vi "HIOKI PW3390 Acquisition Software Trigger.vi"() -> ()   [LabVIEW 2009]
doc: "When each time pushing the trigger button, outputs the specified measurement data."
uses:
  <instrlib>/PW3390/Common/_Initialize/HIOKI PW3390 Initialize LAN.vi
  <instrlib>/PW3390/Common/_Initialize/HIOKI PW3390 Initialize RS-232C.vi
panel:
  out "Selected Item out":string[](array[string])
  in  "Item":T1(array[cluster])=[{"Item"=enum."Urms", "Ch(0:Ch1)"=enum."1"}, {"Item"=enum."Urms", "Ch(0:Ch1)"=enum."2"}, {"Item"=enum."Urms", "Ch(0:Ch1)"=enum."3"}, {"Item"=enum."Urms", "Ch(0:Ch1)"=enum."4"}]
  out "Data out":dbl[](array[numeric])
  out "error out":errorcluster
  in  "Communication Interface":enum16{"LAN", "RS-232C"}(ring)
  in  "COM Port":refnum<visa-resource-name>="COM1"
  in  "baud rate (38400bps)":u32=38400
  in  "IP Address":string="192.168.1.1"
  in  "Trigger":bool
  in  "Stop":bool
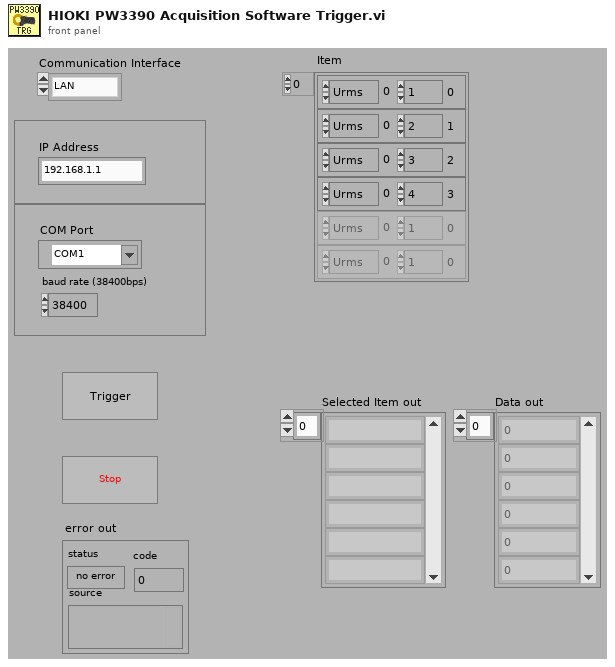
[diagram p1: front panel]
types:
  T1 = cluster{"Item":enum16{"Urms", "Umn", "Uac", "Udc", "Ufnd", "Upk+", "Upk-", "Uthd", "Urf", "Uunb", "Irms", "Imn", "Iac", "Idc", "Ifnd", "Ipk+", "Ipk-", "Ithd", "Irf", "Iunb", "P", "S", "Q", "PF", "DEG U", "DEG I", "DEG P", "f", "EFFI", "LOSS", "IH+", "IH-", "IH", "WP+", "WP-", "WP", "CH A", "CH B", "Pm", "Slip", "Laptime", "Laptime(ms)"}, "Ch(0:Ch1)":enum16{"1", "2", "3", "4", "12", "34", "123"}}[]
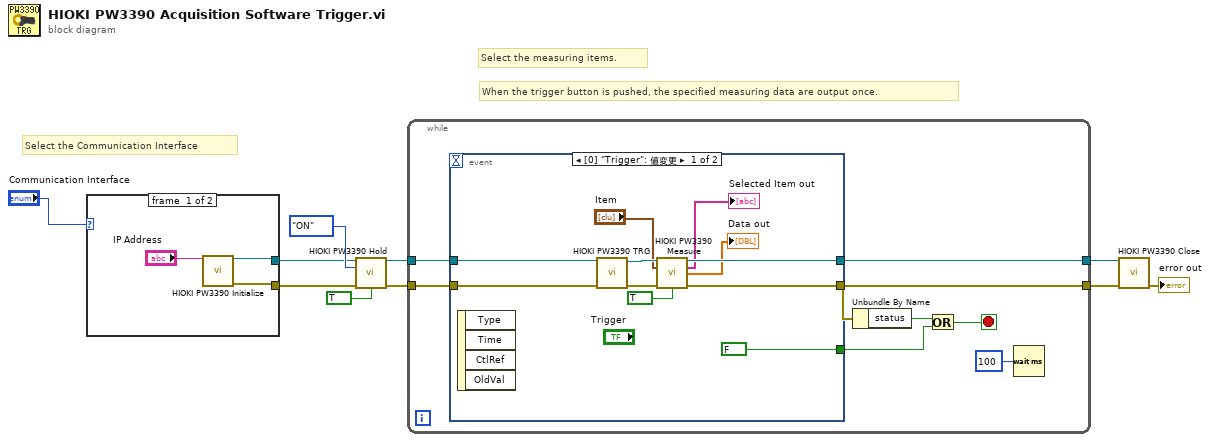
[diagram p0: block diagram]
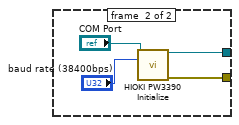
[diagram p2: hidden frame]
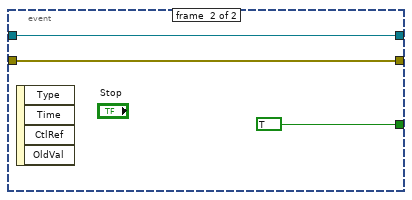
[diagram p3: hidden frame]
diagram:
  # "Select the Communication Interface"
  # "When the trigger button is pushed, the specified measuring data are output once."
  # "Select the measuring items."
  n1 = case shown="\"LAN\", デフォルト" "Communication Interface" {
    tunnel: [w12 w17] -> w4
    tunnel: [w11 w16] -> w3
    frame #0 {
      n2 = call-poly <instrlib>:"HIOKI PW3390 Initialize.vi"("IP Address"="IP Address") -> ("VISA Resource out"=w12:refnum<visa-resource-name>, "error out"=w11:errorcluster)  [unwired: 12 in, 1 out]
    }
    frame #1 {
      n3 = call-poly <instrlib>:"HIOKI PW3390 Initialize.vi"("COM Port"="COM Port", "baud rate (38400bps)"="baud rate (38400bps)") -> ("VISA Resource out"=w17:refnum<visa-resource-name>, "error out"=w16:errorcluster)  [unwired: 11 in, 1 out]
    }
  }
  n4 = call <instrlib>:"HIOKI PW3390 Hold.vi"("VISA Resource"=w4, "HOLD (0: OFF)"=enum16{"OFF", "ON", "PEAK"}."ON", "error in (no error)"=w3, "Error Out (F: Off)"=TRUE) -> ("VISA Resource out"=w8:refnum<visa-resource-name>, "error out"=w7:errorcluster)  [unwired: 9 in, 1 out]
  n5 = while {
    tunnel: [w25] -> w10
    tunnel: [w23] -> w9
    tunnel: w8 -> [w22]
    tunnel: w7 -> [w21]
    stop <- w19 stop-if-true
    n6 = event shown="[0] \"Trigger\": 値変更" {
      selector: _ -> [_ _]
      dyn-events: _ -> [_ _]
      timeout: _ -> [_ _]
      tunnel: [w36 w39] -> w25
      tunnel: [w35 w38] -> w23
      tunnel: w22 -> [w30 w39]
      tunnel: w21 -> [w29 w38]
      tunnel: [FALSE TRUE] -> w18
      event #0 {
        n7 = event-data() -> ()  [unwired: 1 in, 4 out]
        n8 = call <instrlib>:"HIOKI PW3390 TRG.vi"("error in (no error)"=w29, "VISA Resource"=w30) -> ("error out"=w33:errorcluster, "VISA Resource out"=w34:refnum<visa-resource-name>)  [unwired: 8 in]
        n9 = call <instrlib>:"HIOKI PW3390 Measure.vi"("VISA Resource"=w34, "Item"="Item", "error in (no error)"=w33, "Error Out (F: Off)"=TRUE) -> ("VISA Resource out"=w36:refnum<visa-resource-name>, "Selected Item out"=→"Selected Item out":string[], "Data out"=→"Data out":dbl[], "error out"=w35:errorcluster)  [unwired: 6 in, 2 out]
      }
      event #1 {
        n10 = event-data() -> ()  [unwired: 1 in, 4 out]
      }
    }
    n11 = Unbundle By Name(w23) -> ("status"=w20:bool)
    n12 = Or(x=w20, y=w18) -> (x .or. y?=w19:bool)
    n13 = Wait (ms)(milliseconds to wait=u32 100) -> ()  [unwired: 1 out]
  }
  n14 = call <instrlib>:"HIOKI PW3390 Close.vi"("VISA Resource"=w10, "error in (no error)"=w9) -> ("error out"=→"error out":errorcluster)  [unwired: 13 in]
